vi "Signal synchronization sawtooth, square wave, digital output and ramp.vi"() -> ()   [LabVIEW 2020]
doc: "I. Description:\nThis example demonstrates how to continuously output a waveform using an internal sample clock. The automatic regeneration of data has been disabled, so new data has to be provided throughout the duration of the continuous Analog Output operation. This allows the generation of any arbitrary frequency as this VI computes new data for each iteration of the loop, maintaining phase continuity of the signal.\n\nII. Instructions for Running:\n1. Select the Physical Channel to correspond to where your signal is output on the DAQ device.\n2. Enter the Minimum and Maximum Voltage range.\n3. Specify the desired Sample Clock Rate of the output Waveform. Higher sample clock rates will produce a smoother waveform.\n4. Manually specify the Analog Output buffer size, in number of samples. A larger buffer would help non-regenerative operations avoid errors due to occasional high CPU load. \nNote: \nThe Analog Output buffer has to be at least as big as the amount of data being written to the board per iteration. The recommended buffer size would be at least twice the amount of data being written to the board per iteration.\n5. Enter the Waveform Information. See the documentation of the Basic Function Generator SubVI for information on each parameter.\n\nIII. Block Diagram Steps:\n1. Create an Analog Output Voltage channel.\n2. Configure the task to prohibit the automatic regeneration of data.\n3. Call the DAQmx (Sample Clock) VI to set the sample clock rate. Additionally, set the sample mode to Continuous.\n4. Read the actual sample clock rate (eventually coerced depending on the hardware used). \n5. Compute the desired waveform, using the buffer size and the actual update rate. This VI keeps track of the phase of the waveform to ensure that the generated signal is continuous.\n6. Write the waveform to the output buffer. \n7a. Call the Start VI. This is only needed when the loop is executed for the first time.\n7b. Do nothing.\n8. Loop continuously until user presses the Stop button. Every iteration computes and writes a new waveform to the buffer.\n9. Call the Clear Task VI to clear the Task.\n10. Use the popup dialog box to display an error or warning if any.\n\nIV. I/O Connections Overview:\nMake sure your signal output terminal matches the Physical Channel I/O Control. For further connection information, refer to your hardware reference manual."
uses:
  <vilib>/Utility/error.llb/DialogType.ctl
  <vilib>/DAQmx/write.llb/DAQmx Write (Analog 1D Wfm NChan NSamp).vi
  <vilib>/DAQmx/create/channels.llb/DAQmx Create Channel (AO-Voltage-Basic).vi
  <vilib>/DAQmx/create/channels.llb/DAQmx Create Channel (CO-Pulse Generation-Frequency).vi
  <vilib>/DAQmx/configure/timing.llb/DAQmx Timing (Sample Clock).vi
  <vilib>/DAQmx/configure/trigger.llb/DAQmx Start Trigger (Digital Edge).vi
  <vilib>/DAQmx/configure/timing.llb/DAQmx Timing (Implicit).vi
  <vilib>/DAQmx/miscellaneous.llb/DAQmx Fill In Error Info.vi
  <vilib>/measure/NI_MABase.lvlib
  <resource>/objmgr/daqmx.rc
panel:
  out "Number of slices":dbl
  in  "End position (mm)":dbl
  out "last value outside of loop":dbl
  out "Total Z thickness (mm)":dbl
  in  "Z slice width (mm)":dbl
  in  "Start position(mm)":dbl
  in  "square wave duty cycle (%)":dbl=50.0 format="%0.2f"
  in  "Wfm Info":T1(array[cluster]) {"Frequency" format="%.2f"; "Amplitude" format="%0.2p"}
  out "Actual Sample Clock Rate":dbl=20000.0 format="%.2f"
  out "Waveform Graph":waveform(dbl)[](graph) caption="Output Waveform"
  in  "Physical Channels":tag="Dev1/ao0"
  in  "Minimum Value":dbl=-10.0 format="%0.2f"
  in  "Maximum Value":dbl=10.0 format="%0.2f"
  in  "stop":bool
  # "For instructions, select Help>>Show Context Help"
  # "Channel Parameters"
  # "Timing Parameters"
  # "Note:\n\nThe array size should match up with the number of channels in your task.\nEach element in the array will correspond to the settings for a single output channel."
  # "Waveform Information"
  # "Buffer Parameters"
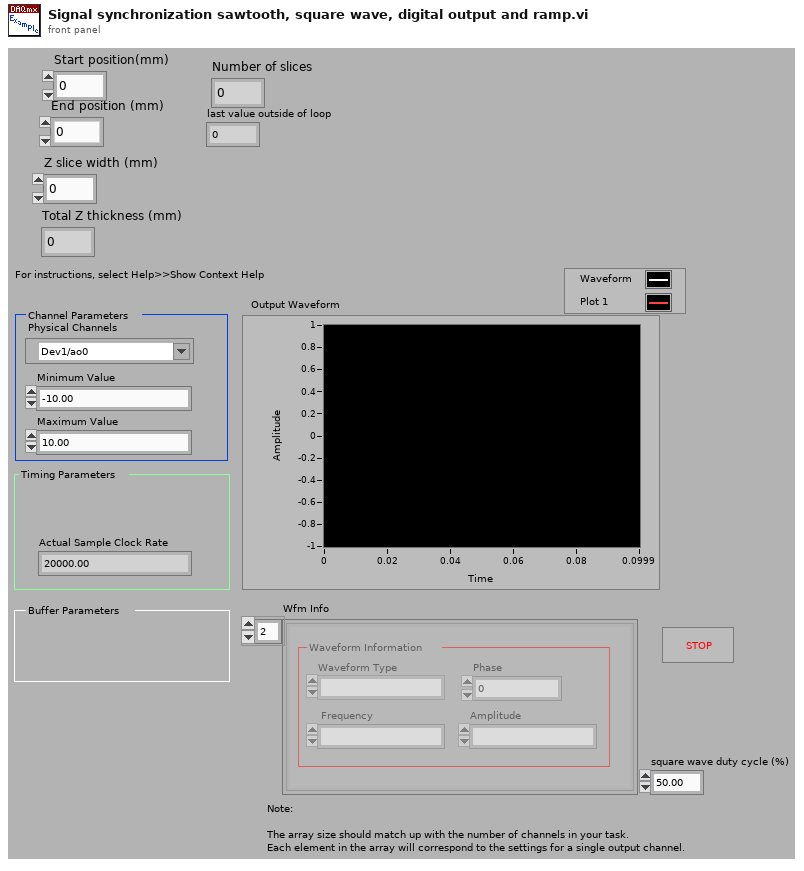
[diagram p1: front panel]
types:
  T1 = cluster{"Waveform Type":enum16{"Sine Wave", "Triangle Wave", "Square Wave", "Sawtooth Wave"}, "Frequency":dbl, "Amplitude":dbl, "Phase":dbl}[]
  T2 = typedef "DialogType.ctl" = u16
  T3 = enum16{"Sine Wave", "Triangle Wave", "Square Wave", "Sawtooth Wave"}
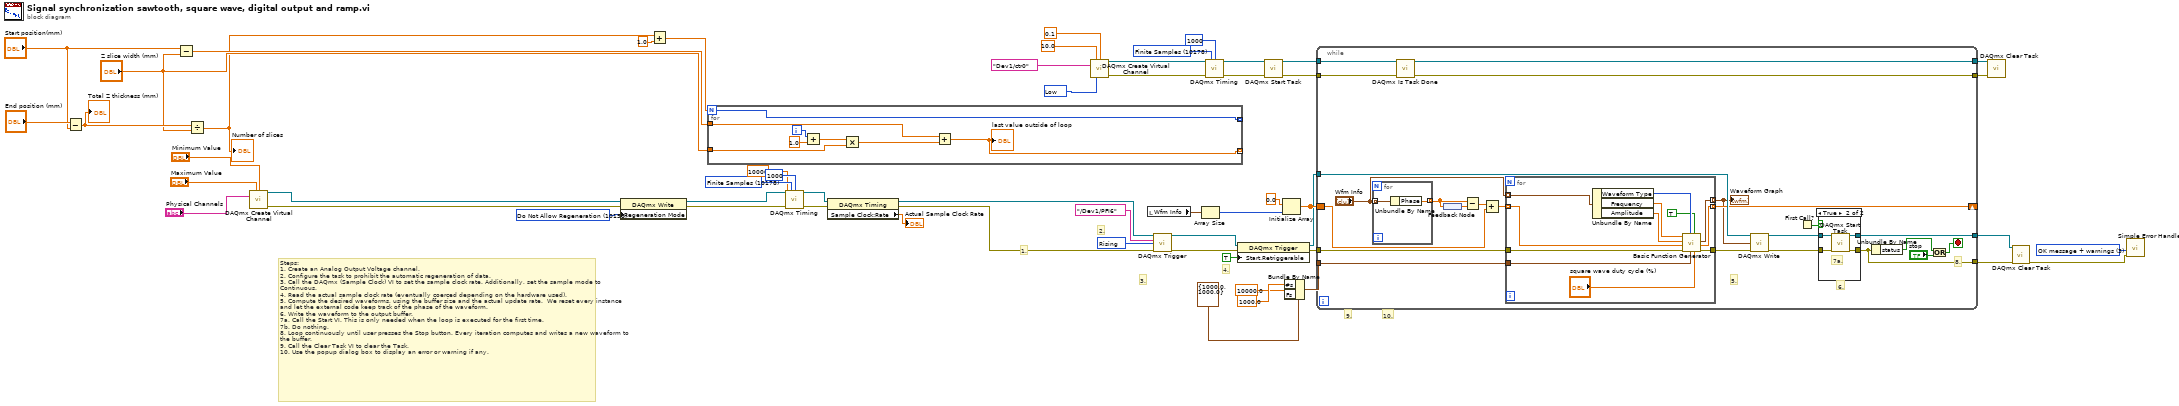
[diagram p0: block diagram]
diagram:
  w15 = 10280 items=["Rising"=10280, "Falling"=10171] ("edge")
  w27 = 10214 items=["High"=10192, "Low"=10214] ("idle state")
  w31 = 10178 items=["Finite Samples"=10178, "Continuous Samples"=10123, "Hardware Timed Single Point"=12522] ("sample mode")
  w44 = 10158 items=["Allow Regeneration"=10097, "Do Not Allow Regeneration"=10158] ("RegenMode")
  w52 = T2 3 items=["no dialog", "OK message", "continue or stop message", "OK message + warnings", "continue/stop + warnings"] ("type of dialog (OK msg:1)")
  w56 = 10178 items=["Finite Samples"=10178, "Continuous Samples"=10123] ("sample mode")
  # "4."
  # "3."
  # "Steps:\n1. Create an Analog Output Voltage channel.\n2. Configure the task to prohibit the automatic regeneration of data.\n3. Call the DAQmx (Sample Clock) VI to set the sample clock rate. Additionally, set the sample mode to Continuous.\n4. Read the actual sample clock rate (eventually coerced depending on the hardware used).\n5. Compute the desired waveforms, using the buffer size and the actual update rate.  We reset every instance and let the external code keep track of the phase of the waveform.\n6. Write the waveform to the output buffer. \n7a. Call the Start VI. This is only needed when the loop is executed for the first time.\n7b. Do nothing.\n8. Loop continuously until user presses the Stop button. Every iteration computes and writes a new waveform to the buffer.\n9. Call the Clear Task VI to clear the Task.\n10. Use the popup dialog box to display an error or warning if any."
  # "10."
  # "9."
  # "2."
  # "1."
  n1 = Subtract(x="End position (mm)", y="Start position(mm)") -> (x-y=w13:dbl)
  "Total Z thickness (mm)" <- w13
  n2 = Subtract(x="Start position(mm)", y="Z slice width (mm)") -> (x-y=w10:dbl)
  n3 = Divide(x=w13, y="Z slice width (mm)") -> (x/y=w6:dbl)
  "Number of slices" <- w6
  n4 = call-poly <vilib>:"DAQmx Create Virtual Channel.vi"("maximum value"="Maximum Value", "minimum value"="Minimum Value", "physical channels"="Physical Channels") -> ("task out"=w43:refnum<k21>, "error out"=w42:errorcluster)  [unwired: 11 in]
  n5 = property class="DAQmx Write"(reference=w43, error in=w42, "Regeneration Mode"=w44) -> (reference out=w41:refnum<k21>, error out=w40:errorcluster)
  n6 = Add(x=w6, y=1.0) -> (x+y=w7:dbl)
  n7 = for {
    N: w7 -> [w58]
    tunnel: w10 -> [w65]
    tunnel: "Z slice width (mm)" -> [w64]
    tunnel: [w62] -> _ mode=indexing
    tunnel: [w58] -> _ mode=indexing
    i -> [w60]
    n8 = Add(x=w60, y=1.0) -> (x+y=w59:dbl)
    n9 = Multiply(x=w59, y=w64) -> (x*y=w63:dbl)
    n10 = Add(x=w65, y=w63) -> (x+y=w62:dbl)
    "last value outside of loop" <- w62
  }
  n11 = call-poly <vilib>:"DAQmx Timing.vi"("task/channels in"=w41, "sample mode"=w56, "samples per channel"=1000, "rate"=10000.0, "error in"=w40) -> ("task out"=w49:refnum<k21>, "error out"=w48:errorcluster)  [unwired: 9 in]
  n12 = property class="DAQmx Timing"(reference=w49, error in=w48) -> (reference out=w17:refnum<k21>, error out=w16:errorcluster, "Sample Clock:Rate"=→"Actual Sample Clock Rate":dbl)
  n13 = call-poly <vilib>:"DAQmx Create Virtual Channel.vi"("frequency"=10.0, "duty cycle"=0.1, "counter"=tag "Dev1/ctr0", "idle state"=w27) -> ("task out"=w32:refnum<k21>, "error out"=w33:errorcluster)  [unwired: 10 in]
  n14 = local read "Wfm Info"() -> (w39:T1)
  n15 = call-poly <vilib>:"DAQmx Trigger.vi"("task/channels in"=w17, "source"=tag "/Dev1/PFI6", "edge"=w15, "error in"=w16) -> ("task out"=w21:refnum<k21>, "error out"=w22:errorcluster)  [unwired: 10 in]
  n16 = Array Size(array=w39) -> (size(s)=w37:i32)
  n17 = call-poly <vilib>:"DAQmx Timing.vi"("task/channels in"=w32, "sample mode"=w31, "samples per channel"=1000, "error in"=w33) -> ("task out"=w34:refnum<k21>, "error out"=w35:errorcluster)  [unwired: 10 in]
  n18 = property class="DAQmx Trigger"(reference=w21, error in=w22, "Start.Retriggerable"=TRUE) -> (reference out=w19:refnum<k21>, error out=w18:errorcluster)
  n19 = call <vilib>:"DAQmx Start Task.vi"("task/channels in"=w34, "error in"=w35) -> ("task out"=w25:refnum<k21>, "error out"=w26:errorcluster)  [unwired: 12 in]
  n20 = Initialize Array(0.0 ("element"), w37) -> (w36:dbl[])
  n21 = Bundle By Name(cluster=cluster{"Fs":dbl, "#s":dbl} {"Fs"=1000.0, "#s"=1000.0} ("sampling info"), "#s"=1000.0, "Fs"=10000.0) -> (w45:cluster{"Fs":dbl, "#s":dbl})
  n22 = while {
    tunnel: w19 -> [w84]
    tunnel: [w80] -> w51
    tunnel: w18 -> [w86]
    tunnel: [w81] -> w50
    tunnel: w45 -> [w78]
    shift-right: [w77] -> _
    shift-left: w36 -> [w73]
    border: w36 -> [_]
    tunnel: [w70] -> w24
    tunnel: [w69] -> w23
    tunnel: w26 -> [w68]
    tunnel: w25 -> [w67]
    stop <- w89 stop-if-true
    # "8."
    # "6."
    # "5."
    n23 = for {
      tunnel: "Wfm Info" -> [w91] mode=indexing
      tunnel: [w90] -> w72 mode=indexing
      n24 = Unbundle By Name(w91) -> ("Phase"=w90:dbl)
    }
    n25 = call <vilib>:"DAQmx Is Task Done.vi"("task/channels in"=w67, "error in"=w68) -> ("task out"=w70:refnum<k21>, "error out"=w69:errorcluster)  [unwired: 11 in, 1 out]
    n26 = feedback-in #1(w72) -> ()
    n27 = feedback #1() -> (w71:dbl[])
    n28 = Subtract(x=w72, y=w71) -> (x-y=w74:dbl[])
    n29 = Add(x=w74, y=w73) -> (x+y=w75:dbl[])
    n30 = for {
      tunnel: w86 -> [w103]
      tunnel: [w102] -> w85
      tunnel: "Wfm Info" -> [w101] mode=indexing
      tunnel: [w97] -> w66 mode=indexing
      tunnel: w78 -> [w96]
      tunnel: [w95] -> w77 mode=indexing
      tunnel: w75 -> [w93] mode=indexing
      n31 = Unbundle By Name(w101) -> ("Waveform Type"=w100:T3, "Frequency"=w99:dbl, "Amplitude"=w98:dbl)
      n32 = call <vilib>:"Basic Function Generator.vi"("square wave duty cycle (%)"="square wave duty cycle (%)", "reset signal"=TRUE, "sampling info"=w96, "signal type"=w100, "error in (no error)"=w103, "phase"=w93, "amplitude"=w98, "frequency"=w99) -> ("error out"=w102:errorcluster, "phase out"=w95:dbl, "signal out"=w97:waveform(dbl))  [unwired: 1 in]
    }
    "Waveform Graph" <- w66
    n33 = call-poly <vilib>:"DAQmx Write.vi"("task/channels in"=w84, "data"=w66, "error in"=w85) -> ("task out"=w83:refnum<k21>, "error out"=w82:errorcluster)  [unwired: 10 in, 1 out]
    n34 = First Call?() -> (First Call?: T/F=w79:bool)
    n35 = case shown="True" w79 {
      tunnel: w83 -> [w105 w109]
      tunnel: w82 -> [w104 w108]
      tunnel: [w104 w107] -> w81
      tunnel: [w105 w106] -> w80
      frame False {
        # "7b."
      }
      frame True {
        # "7a."
        n36 = call <vilib>:"DAQmx Start Task.vi"("task/channels in"=w109, "error in"=w108) -> ("task out"=w106:refnum<k21>, "error out"=w107:errorcluster)  [unwired: 12 in]
      }
    }
    n37 = Unbundle By Name(w81) -> ("status"=w88:bool)
    n38 = Or(x=w88, y="stop") -> (x .or. y?=w89:bool)
  }
  n39 = call <vilib>:"DAQmx Clear Task.vi"("task in"=w24, "error in"=w23) -> ()  [unwired: 13 in, 1 out]
  n40 = call <vilib>:"DAQmx Clear Task.vi"("task in"=w51, "error in"=w50) -> ("error out"=w57:errorcluster)  [unwired: 13 in]
  n41 = call <vilib>:"Simple Error Handler.vi"("type of dialog (OK msg:1)"=w52, "error in (no error)"=w57) -> ()  [unwired: 3 in, 5 out]
